vi "Return Message.vi"(8 "error in (no error)":errorcluster, 9 "Connection ID":string, 10 "Message To Return":refnum<class "IPacket.lvclass">, 11 "HeaderDataPacketReturn in":refnum<class "Header Data Packet Return.lvclass">) -> (0 "error out":errorcluster)   [LabVIEW 2020, in "Network Messenger.lvlib" / "Header Data Packet Return.lvclass"]
uses:
  <vilib>/gpm_packages/@cs/Network-interface/Source/Network Messenger/Header Data Packet Return/Header Data Packet Return.lvclass
  <vilib>/gpm_packages/@cs/Network-interface/Source/MessagingInterfaces/IPacket/IPacket.lvclass
  <vilib>/gpm_packages/@cs/Network-interface/Source/Network Messenger/ClusterMessagePacket/ClusterMessagePacket.lvclass
  <vilib>/gpm_packages/@cs/Network-interface/Source/Network Messenger/Header Data Packet Return/Header Data Packet Return.lvclass/Header Data Packet Return.ctl
  <vilib>/gpm_packages/@cs/Network-interface/Source/Network Messenger/IPacket Return/IPacket Return.lvclass
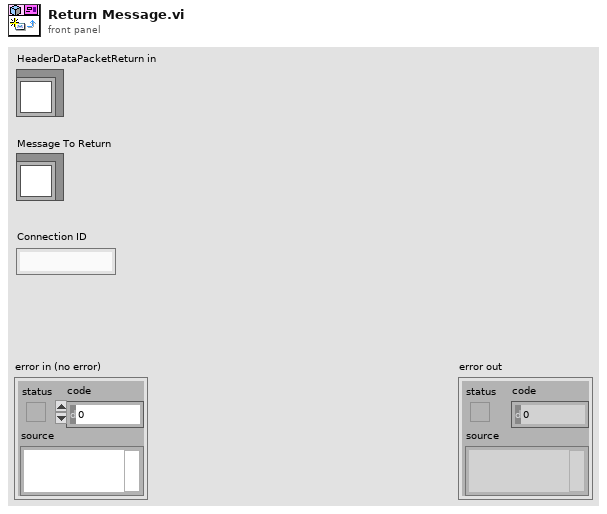
[diagram p1: front panel]
types:
  T1 = typedef "Network Messenger.lvlib/Message Packet.ctl" = cluster{"Msg":string, "Data":variant}
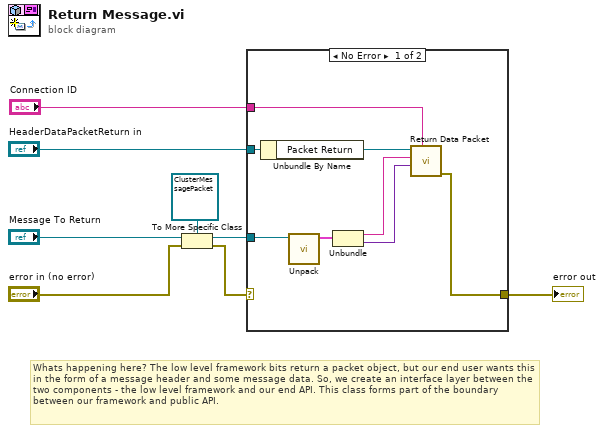
[diagram p0: block diagram]
diagram:
  # "Whats happening here? The low level framework bits return a packet object, but our end user wants this in the form of a message header and some message data. So, we create an interface layer between the two components - the low level framework and our end API. This class forms part of the boundary between our framework and public API."
  n1 = To More Specific Class(target class=refnum<class "ClusterMessagePacket.lvclass"> refnum ("Network Messenger.lvlib:ClusterMessagePacket.lvclass"), reference="Message To Return", error in="error in (no error)") -> (specific class reference=w4:refnum<class "ClusterMessagePacket.lvclass">, error out=w5:errorcluster)
  n2 = case shown="No Error" w5 {
    selector: w5 -> [_ w17]
    tunnel: w4 -> [w15 _]
    tunnel: "HeaderDataPacketReturn in" -> [w16 _]
    tunnel: [w10 w17] -> w2
    tunnel: "Connection ID" -> [w9 _]
    frame No Error {
      n3 = Unbundle By Name(w16) -> ("Packet Return"=w14:refnum<class "IPacket Return.lvclass">)
      n4 = call <vilib>:"Unpack.vi"("ClusterMessagePacket"=w15) -> ("Packet"=w13:T1)  [unwired: 10 in]
      n5 = Unbundle(w13) -> ("Msg"=w12:string, "Data"=w11:variant)
      n6 = call-dynamic "Return Data Packet.vi"("Connection ID"=w9, "Packet Data"=w11, "Packet Header"=w12, "IPacketReturn in"=w14) -> ("error out"=w10:errorcluster)  [unwired: 7 in]
    }
    frame Error {
      # "I don't think its possible for this to happen based on access scoping.."
    }
  }
  "error out" <- w2
